vi "main_ctrl.vi"(8 "error in":errorcluster) -> (0 "error out":errorcluster caption="Error Out")   [LabVIEW 2013]
uses:
  <vilib>/Rock Robotics/WPI/DriverStation/WPI_DriverStationRobotMode2.ctl
  typedefs/fg_typedef.ctl
  <vilib>/Rock Robotics/WPI/Solenoid/WPI_SolenoidValue.ctl
  typedefs/subStates.ctl
  typedefs/singleUseSubstate.ctl
  typedefs/vision enable.ctl
  <vilib>/Rock Robotics/WPI/Compressor/WPI_CompressorGetSetRefNum.vi
  <vilib>/Rock Robotics/WPI/RobotDrive/WPI_RobotDriveGetSetRefNum.vi
  <vilib>/Rock Robotics/WPI/Solenoid/WPI_SolenoidGetEnum.vi
  <vilib>/Rock Robotics/WPI/Solenoid/WPI_SolenoidSetEnum.vi
  <vilib>/Rock Robotics/WPI/RobotDrive/WPI_RobotDriveArcadeDrive_Standard(NoSaturation).vi
  typedefs/vision data.ctl
panel:
  in  "Arcade Drive?":bool=TRUE
  out "Y Axis":dbl
  out "X Axis":dbl
  out "error In":errorcluster caption="Error In"
  out "Belts":dbl(knob) scale=-1.0..1.0
  out "Arm Encoder Rate":dbl(graph)
  out "Arm Encoder Distance":dbl(graph)
  out "Shifter State":cluster{"Shifted High":bool, "Shifted Low":bool}
  out "Extended":bool
  out "Retracted":bool
  out "Light Sensor":bool
  out "Belt Output":dbl
  out "Arm Distance":dbl
  out "Arm Rate":dbl
  in  "Joystick Override":bool
  in  "Joystick Y Manual":dbl(slide) scale=-1.0..1.0
  out "Left Drive Distance":dbl
  out "Right Drive Distance":dbl
  out "Left Drive Rate":dbl
  out "Right Drive Rate":dbl
  in  "Piston Actuation Commands":T1
  in  "Enables":T2
  out "Robot Mode":T3
  out "Vision SPI":u32
  out "Vision IPS":dbl
  out "Main IPS":dbl
  out "Main SPI":u32
  # "Inputs"
  # "Sensors"
  # "MAIN CONTROL"
  # "holds robot control code - dual parallel state machine"
  # "SPI: milliseconds per iteration\nIPS: iterations per second"
  # "Right Shooter Piston Sensors"
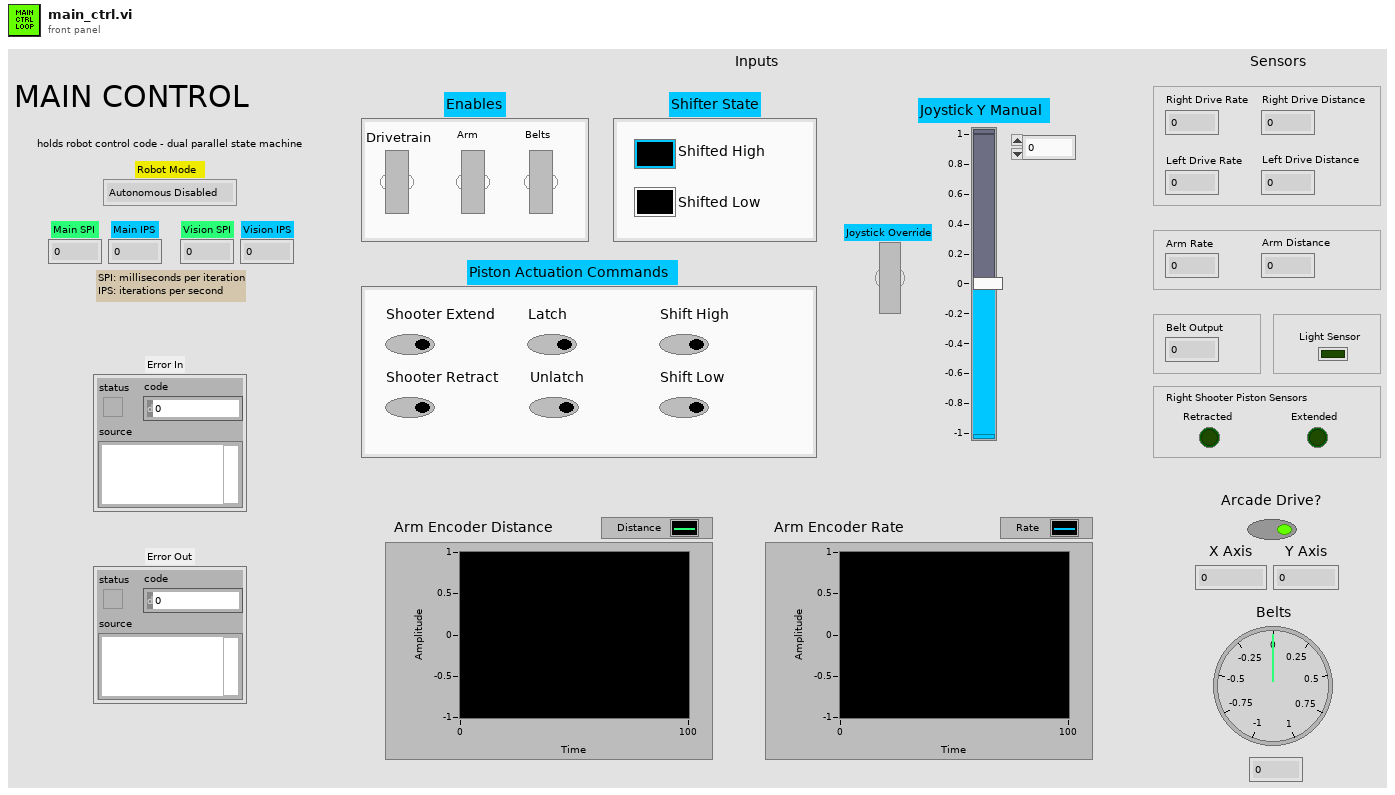
[diagram p1: front panel]
types:
  T1 = cluster{"Shooter Extend":bool, "Shooter Retract":bool, "Latch":bool, "Unlatch":bool, "Shift High":bool, "Shift Low":bool}
  T2 = cluster{"Drivetrain":bool, "Arm":bool, "Belts":bool}
  T3 = typedef "WPI_DriverStationRobotMode2.ctl" = enum16{"Autonomous Disabled", "Autonomous Enabled", "Teleop Disabled", "Teleop Enabled", "Timeout", "Finish", "Test Disabled", "Test Enabled"}
  T4 = typedef "WPI_RobotDriveDevRef.ctl" = cluster{"DevStatus":errorcluster, "Motors[]":T5[], "Square Inputs":bool, "Max Output":dbl, "Isochronous":bool}
  T5 = typedef "WPI_MotorControlDeviceRef.ctl" = cluster{"DeviceStatus":errorcluster, "Type":enum16{"PWM", "CAN"}, "PWM":cluster{"Digital Module":T6, "PWM Channel":T7, "DeadBand":T8}, "CAN":cluster{"Device Number":u8, "Control Mode":T9, "Semaphore":T10, "Max Vout":dbl}, "Invert":bool, "TransformRef":T11, "InvTransformRef":T11}
  T6 = typedef "FPGA_TypedefDigitalModule.ctl" = enum16{"Digital Module 1", "Digital Module 2"}
  T7 = typedef "FPGA_DIOPWMChannel.ctl" = enum8{"PWM 1", "PWM 2", "PWM 3", "PWM 4", "PWM 5", "PWM 6", "PWM 7", "PWM 8", "PWM 9", "PWM 10", "Invalid"}
  T8 = typedef "WPI_PWMDeadband.ctl" = cluster{"Name":string, "maxPositivePwm":i32, "minPositivePwm":i32, "centerPwm":i32, "maxNegativePwm":i32, "minNegativePwm":i32, "angularRange":u16}
  T9 = typedef "WPI_CANJaguar_ControlMode.ctl" = enum8{"Percent VBus", "Current", "Speed", "Position", "Voltage"}
  T10 = typedef "Semaphore RefNum" = refnum<k1>
  T11 = typedef "WPI_PWMTransform_ConPane.ctl" = refnum<vi>
  T12 = typedef "WPI_SolenoidDevRef.ctl" = cluster{"DevStatus":errorcluster, "Solenoid Module":T13, "Forward Solenoid Channel":T14, "Reverse Solenoid Channel":T14}
  T13 = typedef "FPGA_TypedefSolenoidModule.ctl" = enum16{"Solenoid Module 1", "Solenoid Module 2"}
  T14 = typedef "WPI_SolenoidChannel.ctl" = enum8{"Solenoid 1", "Solenoid 2", "Solenoid 3", "Solenoid 4", "Solenoid 5", "Solenoid 6", "Solenoid 7", "Solenoid 8", "Invalid"}
  T15 = typedef "WPI_CompressorDevRef.ctl" = cluster{"DevStatus":errorcluster, "DigitalInputDevRef":T16, "RelayDevRef":T18}
  T16 = typedef "WPI_DigitalInputDevRef.ctl" = cluster{"DevStatus":errorcluster, "DIO Channel":T17, "Digital Module":T6}
  T17 = typedef "FPGA_DIOChannel.ctl" = enum8{"DIO 1", "DIO 2", "DIO 3", "DIO 4", "DIO 5", "DIO 6", "DIO 7", "DIO 8", "DIO 9", "DIO 10", "DIO 11", "DIO 12", "DIO 13", "DIO 14", "Invalid"}
  T18 = typedef "WPI_RelayDevRef.ctl" = cluster{"DevStatus":errorcluster, "Relay Channel":T19, "Digital Module":T6, "Relay Direction":T20}
  T19 = typedef "FPGA_DIORelayChannel.ctl" = enum8{"Relay 1", "Relay 2", "Relay 3", "Relay 4", "Relay 5", "Relay 6", "Relay 7", "Relay 8", "Invalid"}
  T20 = typedef "WPI_RelayDirection.ctl" = enum16{"Both directions", "Forward only", "Reverse only"}
  T21 = typedef "vision data.ctl" = cluster{"x":dbl, "y":dbl, "area":dbl, "width":dbl, "height":dbl, "Hot Goal Present?":bool, "distance":dbl}
  T22 = typedef "vision enable.ctl" = enum16{"Enable", "Disable", "Stop"}
  T23 = typedef "fg_typedef.ctl" = enum16{"Get", "Set"}
  T24 = typedef "WPI_CameraDevRef.ctl" = cluster{"Camera Address":string, "CameraStatus":errorcluster, "Acquire Image Notifier":refnum<notifier>}
  T25 = typedef "IMAQ Image.ctl" = refnum<image>
  T26 = cluster{"Vision mSPI":u32, "Main mSPI":u32, "Dash mSPI":u32}
  T27 = typedef "WPI_SolenoidValue.ctl" = enum16{"Off", "On", "Forward", "Reverse"}
  T28 = typedef "singleUseSubstate.ctl" = enum16{"null", "wait", "shift high", "shift low"}
  T29 = cluster{"Joystick Y Manual":dbl, "Joystick Override":bool, "Piston Actuation Commands":cluster{"Shooter Extend":bool, "Shooter Retract":bool, "Latch Extend":bool, "Latch Retract":bool, "Shift High":bool, "Shift Low":bool}, "Enables":cluster{"Drivetrain":bool, "Arm":bool, "Belts":bool}}
  T30 = typedef "WPI_DriverStationDerivedRobotMode.ctl" = enum16{"Init", "Execute", "Stop"}
  T31 = typedef "subStates.ctl" = enum16{"null", "wait", "driver control", "auto", "manual override", "hold position", "rotate", "pickup", "pass", "load", "goto shoot", "shoot", "cancel", "end"}
  T32 = typedef "Loop 2 Datatype.ctl" = cluster{"State":T31, "Waiting Loop":i32, "State to Wait For":i32, "Loop ID":i32, "Exit Value":i32, "Joystick Y":dbl}
  T33 = typedef "Loop 1 Datatype.ctl" = cluster{"State":T31, "Waiting Loop":i32, "State to Wait For":i32, "Loop ID":i32, "Exit Value":i32}
  T34 = typedef "Loop 3 Datatype.ctl" = cluster{"State":T31, "Waiting Loop":i32, "State to Wait For":i32, "Loop ID":i32, "Exit Value":i32, "Joystick Y":dbl}
  T35 = typedef "Loop 0 Datatype.ctl" = cluster{"State":T31, "Waiting Loop":i32, "State to Wait For":i32, "Loop ID":i32, "Exit Value":i32, "X Axis":dbl, "Y Axis":dbl}
  T36 = typedef "Loop 4 Datatype.ctl" = cluster{"State":T31, "Waiting Loop":i32, "State to Wait For":i32, "Loop ID":i32, "Exit Value":i32}
  T37 = typedef "WPI_EncoderDevRef.ctl" = cluster{"DevStatus":errorcluster, "EncoderIndex":T38, "CounterIndex":T39, "DistancePerCount":dbl, "Decoding Type":T40}
  T38 = typedef "FPGA_EncoderIdx.ctl" = enum8{"Enc 0", "Enc 1", "Enc 2", "Enc 3", "Invalid"}
  T39 = typedef "FPGA_CounterCtrSystemIndex.ctl" = enum8{"Ctr 0", "Ctr 1", "Ctr 2", "Ctr 3", "Ctr 4", "Ctr 5", "Ctr 6", "Ctr 7", "Invalid"}
  T40 = typedef "WPI_EncoderType.ctl" = enum16{"1x", "2x", "4x"}
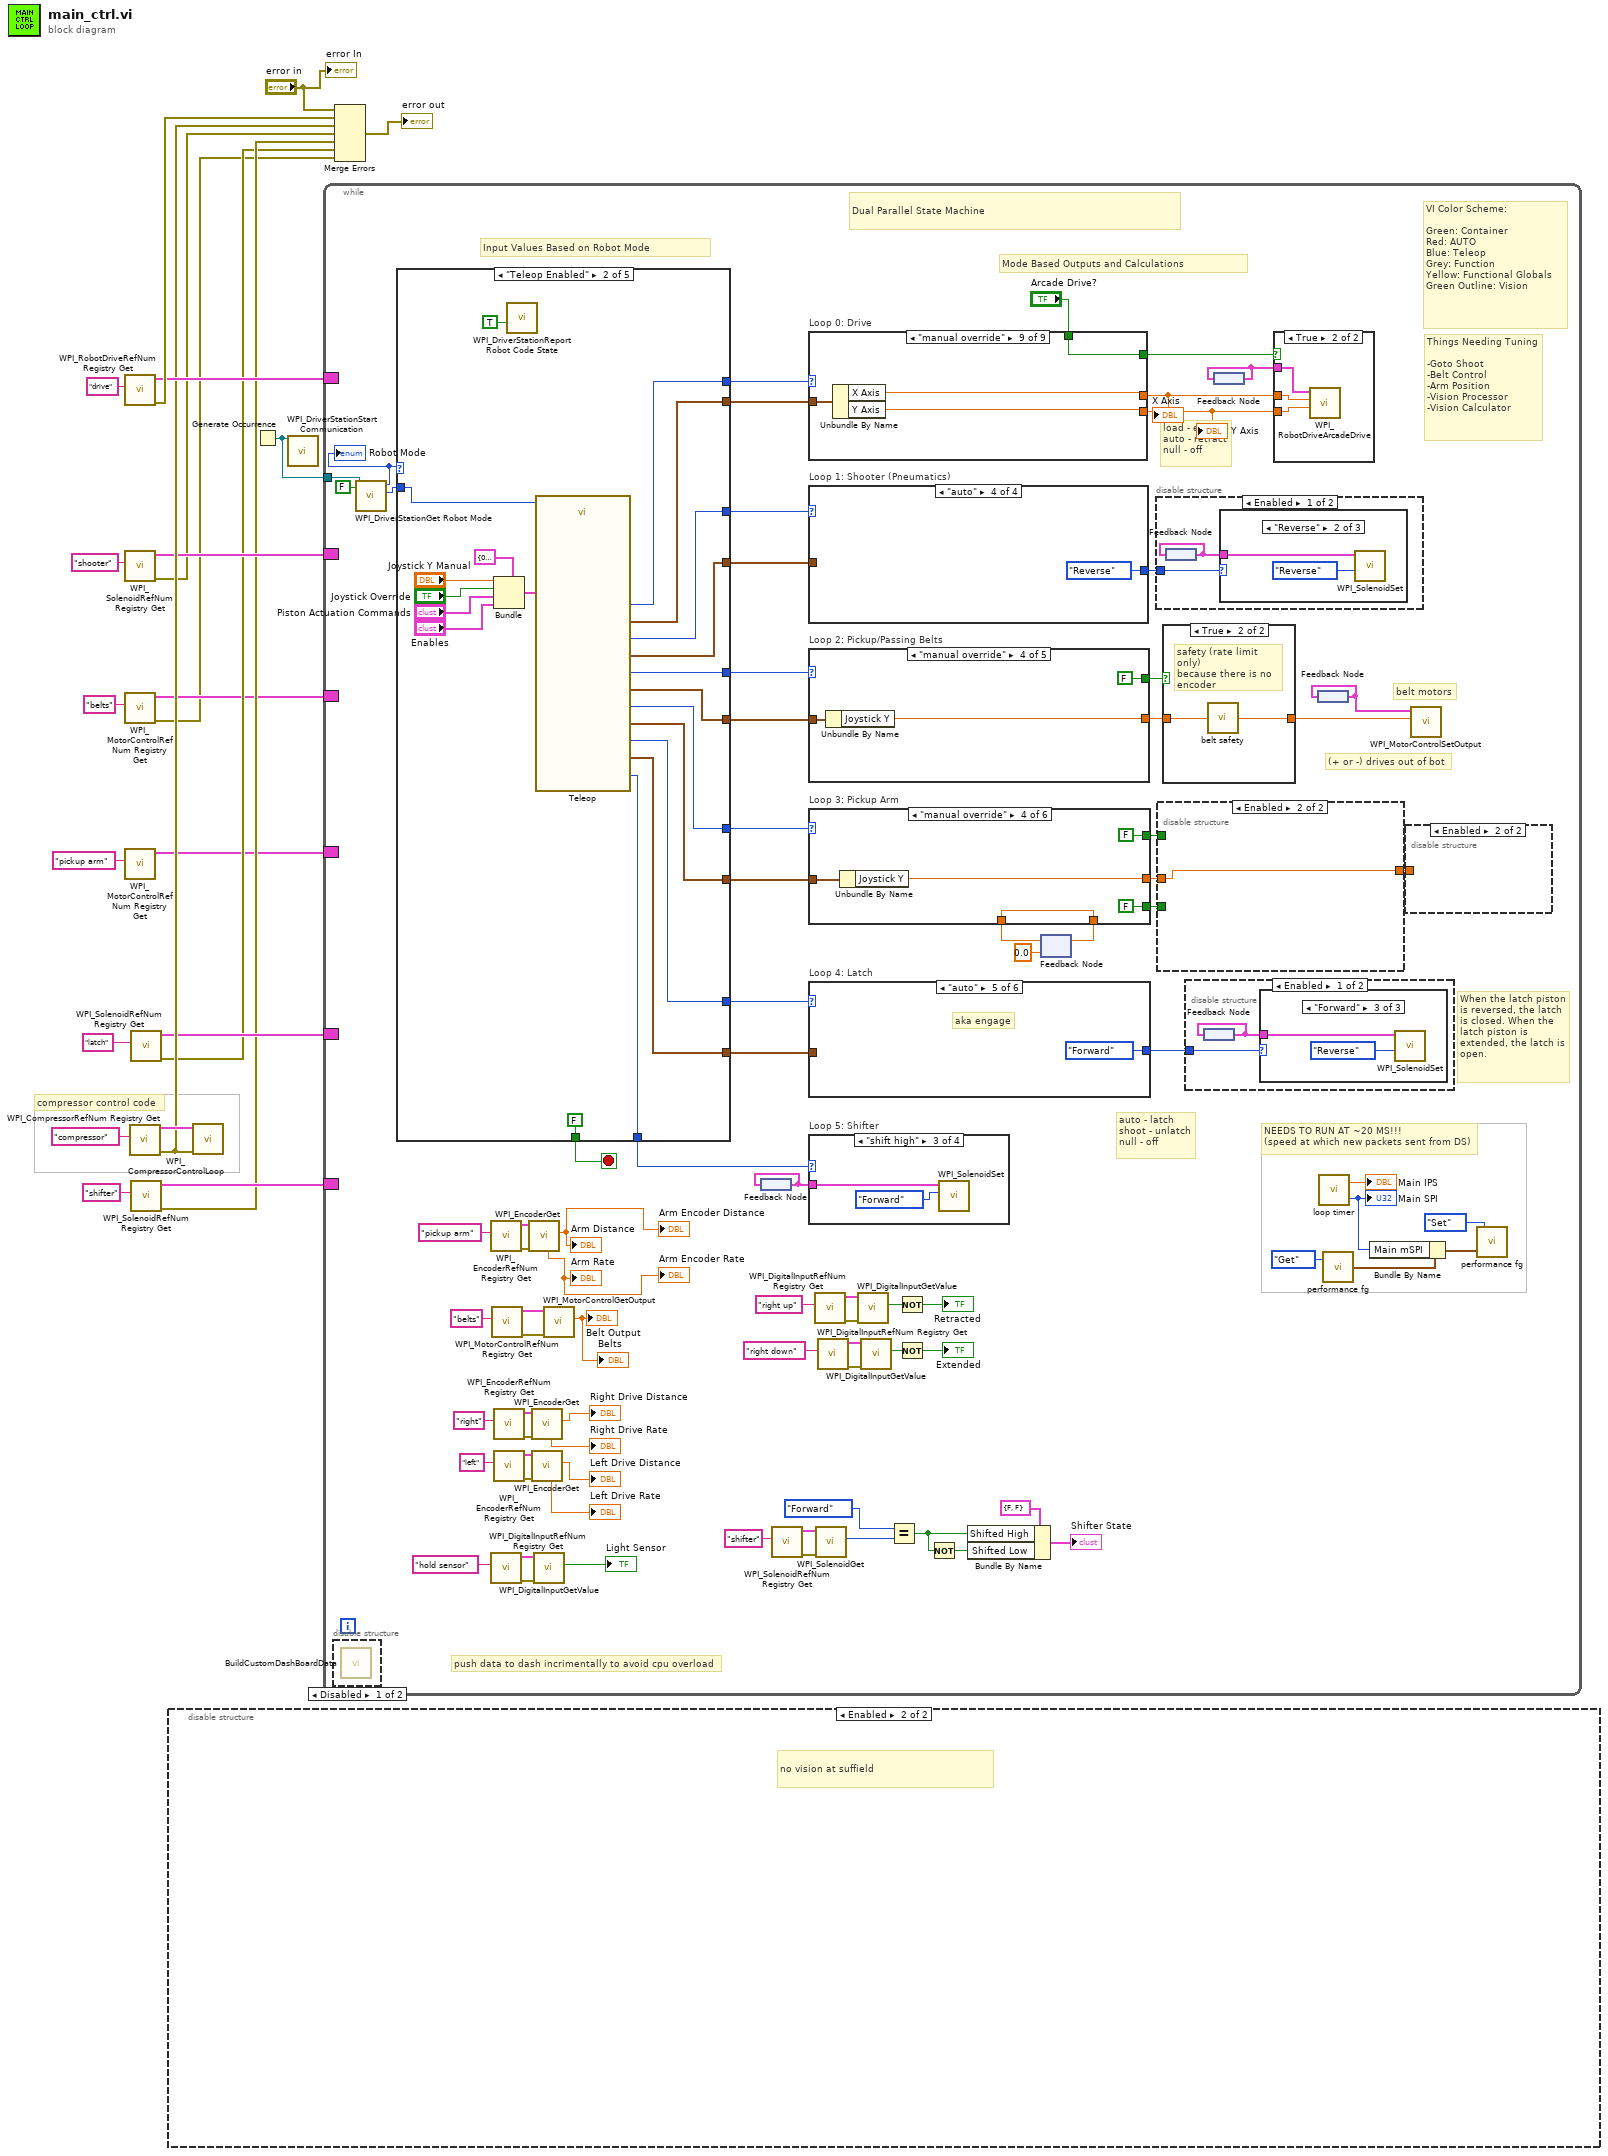
[diagram p0: block diagram]
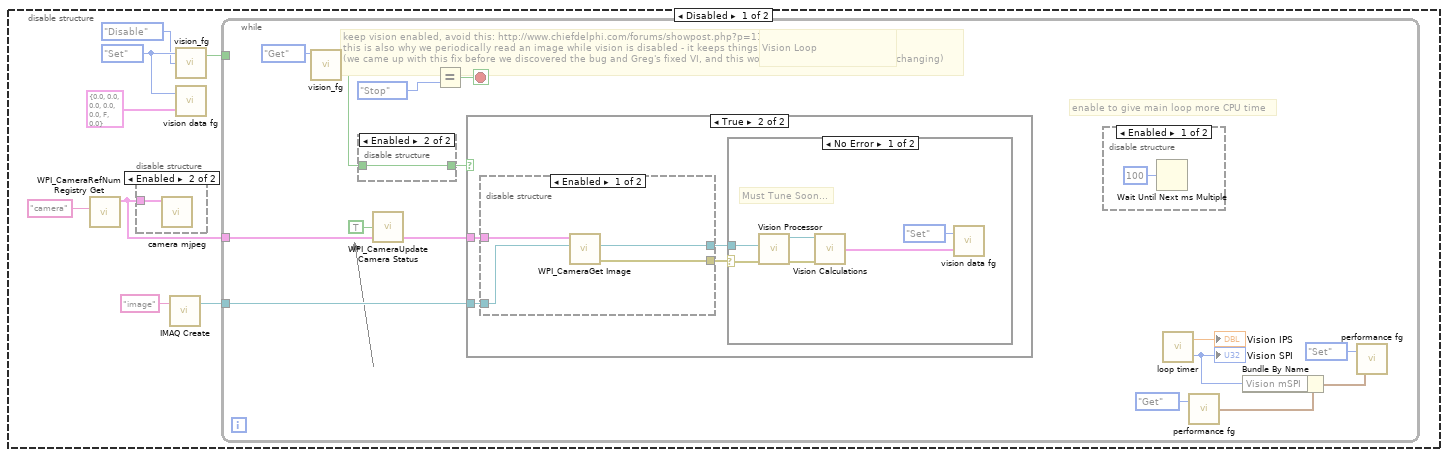
[diagram p2: hidden frame]
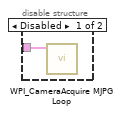
[diagram p3: hidden frame]
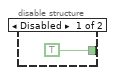
[diagram p4: hidden frame]
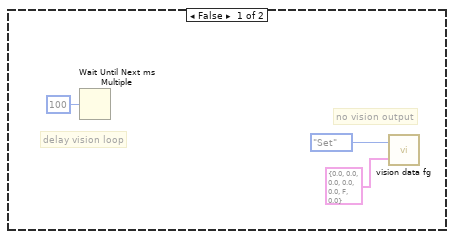
[diagram p6: hidden frame]
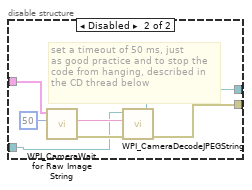
[diagram p8: hidden frame]
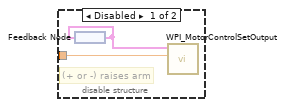
[diagram p10: hidden frame]
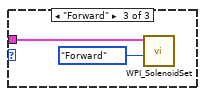
[diagram p12: hidden frame]
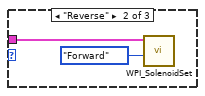
[diagram p15: hidden frame]
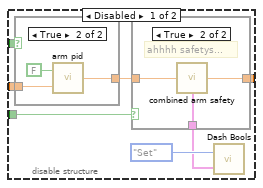
[diagram p17: hidden frame]
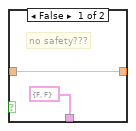
[diagram p18: hidden frame]
diagram:
  # "compressor control code"
  n1 = call <vilib>:"WPI_RobotDriveRefNum Registry Get.vi"("refnum name"="drive") -> ("error out"=w20:errorcluster, "RobotDriveDevRef"=w19:T4)  [unwired: 9 in]
  n2 = call <vilib>:"WPI_SolenoidRefNum Registry Get.vi"("refnum name"="shooter") -> ("error out"=w8:errorcluster, "SolenoidDevRef"=w12:T12)  [unwired: 9 in]
  n3 = call <vilib>:"WPI_MotorControlRefNum Registry Get.vi"("refnum name"="belts") -> ("error out"=w4:errorcluster, "MotorControlDevRef"=w6:T5)  [unwired: 9 in]
  n4 = call <vilib>:"WPI_MotorControlRefNum Registry Get.vi"("refnum name"="pickup arm") -> ("MotorControlDevRef"=w2:T5)  [unwired: 9 in, 1 out]
  n5 = call <vilib>:"WPI_CompressorRefNum Registry Get.vi"("refnum name"="compressor") -> ("error out"=w15:errorcluster, "CompressorDevRef"=w18:T15)  [unwired: 9 in]
  n6 = call <vilib>:"WPI_SolenoidRefNum Registry Get.vi"("refnum name"="latch") -> ("error out"=w7:errorcluster, "SolenoidDevRef"=w10:T12)  [unwired: 9 in]
  n7 = call <vilib>:"WPI_SolenoidRefNum Registry Get.vi"("refnum name"="shifter") -> ("error out"=w9:errorcluster, "SolenoidDevRef"=w17:T12)  [unwired: 9 in]
  n8 = disable-structure shown="Enabled" {
    frame Disabled {
      w29 = fg_typedef."Set" ("Enum")
      n9 = call <vilib>:"WPI_CameraRefNum Registry Get.vi"("refnum name"="camera") -> ("CameraDevRef"=w26:T24)  [unwired: 9 in, 1 out]
      n10 = disable-structure shown="Enabled" {
        disable-tunnel: w26 -> [w32 w33]
        frame Disabled {
          n11 = call <vilib>:"WPI_CameraAcquire MJPG Loop.vi"("CameraDevRef"=w32) -> ()  [unwired: 11 in]
        }
        frame Enabled {
          n12 = call "camera mjpeg.vi"("CameraDevRef"=w33) -> ()  [unwired: 11 in]
        }
      }
      n13 = call "IMAQ Create"("Image Name"="image") -> ("New Image"=w31:T25)  [unwired: 4 in, 1 out]
      n14 = call "vision_fg.vi"("Action"=vision_enable."Disable", "Menu"=w29) -> ("Enabled?"=w30:bool)  [unwired: 1 in, 1 out]
      n15 = call "vision data fg.vi"("Input"=T21 {"x"=0.0, "y"=0.0, "area"=0.0, "width"=0.0, "height"=0.0, "Hot Goal Present?"=FALSE, "distance"=0.0} ("Cluster"), "Menu"=w29) -> ()  [unwired: 1 out]
      n16 = while {
        tunnel: w31 -> [w48]
        tunnel: w26 -> [w47]
        tunnel: w30 -> [_]
        stop <- w49 stop-if-true
        # "keep vision enabled, avoid this: http://www.chiefdelphi.com/forums/showpost.php?p=1128407&postcount=2\nthis is also why we periodically read an image while vision is disabled - it keeps things from timing out\n(we came up with this fix before we discovered the bug and Greg's fixed VI, and this worked well, so it wasn't worth changing)"
        # "enable to give main loop more CPU time"
        # "Vision Loop"
        n17 = call "vision_fg.vi"("Menu"=fg_typedef."Get" ("Enum")) -> ("State Out"=w43:T22, "Enabled?"=w34:bool)  [unwired: 2 in]
        n18 = disable-structure shown="Enabled" {
          disable-tunnel: [TRUE w51] -> w35
          disable-tunnel: w34 -> [_ w51]
          frame Disabled {
          }
          frame Enabled {
          }
        }
        n19 = call <vilib>:"WPI_CameraUpdate Camera Status.vi"("CameraDevRef In"=w47, "Enable Vision"=TRUE) -> ("CameraDevRef Out"=w46:T24)  [unwired: 3 in]
        n20 = Equal?(x=w43, y=vision_enable."Stop") -> (x = y?=w49:bool)
        n21 = case shown="True" w35 {
          tunnel: w48 -> [_ w59]
          tunnel: w46 -> [_ w58]
          frame False {
            # "no vision output"
            # "delay vision loop"
            n22 = Wait Until Next ms Multiple(millisecond multiple=u32 100) -> ()  [unwired: 1 out]
            n23 = call "vision data fg.vi"("Input"=T21 {"x"=0.0, "y"=0.0, "area"=0.0, "width"=0.0, "height"=0.0, "Hot Goal Present?"=FALSE, "distance"=0.0} ("Cluster"), "Menu"=fg_typedef."Set" ("Enum")) -> ()  [unwired: 1 out]
          }
          frame True {
            n24 = disable-structure shown="Enabled" {
              disable-tunnel: w59 -> [w68 w72]
              disable-tunnel: w58 -> [w69 w74]
              disable-tunnel: [w67 w71] -> w57
              disable-tunnel: [w66 w70] -> w56
              frame Enabled {
                n25 = call <vilib>:"WPI_CameraGet Image.vi"("Image"=w68, "CameraDevRef"=w69) -> ("error out"=w66:errorcluster, "Image Out"=w67:T25)  [unwired: 7 in, 1 out]
              }
              frame Disabled {
                # "set a timeout of 50 ms, just\nas good practice and to stop the \ncode from hanging, described in \nthe CD thread below"
                n26 = call <vilib>:"WPI_CameraWait for Raw Image String.vi"("Timeout in ms (-1)"=50, "CameraDevRef"=w74) -> ("error out"=w76:errorcluster, "String"=w75:string)  [unwired: 3 in, 5 out]
                n27 = call <vilib>:"WPI_CameraDecodeJPEGString.vi"("error in"=w76, "Compressed Image"=w75, "Image In"=w72) -> ("error out"=w70:errorcluster, "Image Out"=w71:T25)  [unwired: 3 out]
              }
            }
            n28 = case shown="No Error" w56 {
              selector: w56 -> [w64 _]
              tunnel: w57 -> [w63 _]
              frame No Error {
                # "Must Tune Soon..."
                n29 = call "Vision Processor.vi"("error in"=w64, "Image In"=w63) -> ("error out"=w61:errorcluster, "Image Out"=w62:T25)  [unwired: 5 in]
                n30 = call "Vision Calculations.vi"("Image In"=w62, "error in"=w61) -> ("Vision Data"=w60:T21)  [unwired: 3 in]
                n31 = call "vision data fg.vi"("Input"=w60, "Menu"=fg_typedef."Set" ("Enum")) -> ()  [unwired: 1 out]
              }
              frame Error {
              }
            }
          }
        }
        n32 = disable-structure shown="Enabled" {
          frame Enabled {
            n33 = Wait Until Next ms Multiple(millisecond multiple=u32 100) -> ()  [unwired: 1 out]
          }
          frame Disabled {
          }
        }
        n34 = call "loop timer.vi"() -> ("IPS"=→"Vision IPS":dbl, "SPI"=w41:u32)  [unwired: 1 in]
        "Vision SPI" <- w41
        n35 = call "performance fg.vi"("Menu"=fg_typedef."Get") -> ("Output"=w39:T26)  [unwired: 1 in]
        n36 = Bundle By Name(cluster=w39, "Vision mSPI"=w41) -> (w38:T26)
        n37 = call "performance fg.vi"("Input"=w38, "Menu"=fg_typedef."Set") -> ()  [unwired: 1 out]
      }
    }
    frame Enabled {
      # "no vision at suffield"
    }
  }
  n38 = call <vilib>:"WPI_CompressorControlLoop.vi"("error in (no error)"=w15, "CompressorDevRef"=w18) -> ()  [unwired: 10 in]
  n39 = Generate Occurrence() -> (w14:refnum<k4>)
  n40 = call <vilib>:"WPI_DriverStationStart Communication.vi"("occurrence"=w14) -> ()  [unwired: 11 in]
  n41 = while {
    tunnel: w14 -> [w82]
    border: w19 -> [_]
    border: w17 -> [_]
    border: w12 -> [_]
    border: w10 -> [_]
    border: w6 -> [_]
    border: w2 -> [_]
    stop <- w156 stop-if-true
    # "belt motors"
    # "auto - latch\nshoot - unlatch\nnull - off"
    # "load - extend\nauto - retract\nnull - off"
    # "When the latch piston\nis reversed, the latch\nis closed. When the\nlatch piston is\nextended, the latch is\nopen."
    # "push data to dash incrimentally to avoid cpu overload"
    # "Things Needing Tuning\n\n-Goto Shoot\n-Belt Control\n-Arm Position\n-Vision Processor\n-Vision Calculator"
    # "(+ or -) drives out of bot"
    # "VI Color Scheme:\n\nGreen: Container\nRed: AUTO\nBlue: Teleop\nGrey: Function\nYellow: Functional Globals\nGreen Outline: Vision"
    # "Input Values Based on Robot Mode"
    # "Mode Based Outputs and Calculations"
    # "NEEDS TO RUN AT ~20 MS!!!\n(speed at which new packets sent from DS)"
    # "Dual Parallel State Machine"
    n42 = disable-structure shown="Disabled" {
      frame Disabled {
        n43 = call "BuildCustomDashBoardData.vi"() -> ()  [unwired: 12 in]
      }
      frame Enabled {
      }
    }
    n44 = call <vilib>:"WPI_DriverStationGet Robot Mode.vi"("Finish"=FALSE, "DS Occurrence"=w82) -> ("Call Context"=w80:T30, "Robot Mode"=w81:T3)  [unwired: 8 out]
    "Robot Mode" <- w81
    n45 = case shown="\"Teleop Enabled\"" w81 {
      tunnel: [w369 w406 w408 w414 w420] -> w137
      tunnel: w80 -> [w360 w402 _ _ _]
      tunnel: [w367 w405 w408 w414 w420] -> w158
      tunnel: [w361 w403 singleUseSubstate."null" ("SubState 5") singleUseSubstate."null" ("SubState 5") singleUseSubstate."null" ("SubState 5")] -> w157
      tunnel: [FALSE FALSE FALSE FALSE TRUE] -> w156
      tunnel: [w371 w401 w408 w414 w420] -> w149
      tunnel: [w370 w400 _ _ _] -> w150
      tunnel: [w368 w399 _ _ _] -> w148
      tunnel: [w366 w398 _ _ _] -> w147
      tunnel: [w364 w397 _ _ _] -> w145
      tunnel: [w362 w396 _ _ _] -> w144
      tunnel: [w363 w395 w408 w414 w420] -> w143
      tunnel: [w365 w394 w408 w414 w420] -> w142
      frame "Autonomous Enabled" {
        n46 = disable-structure shown="Enabled" {
          disable-tunnel: [w384 w386] -> w371
          disable-tunnel: [w383 _] -> w370
          disable-tunnel: [w382 w386] -> w369
          disable-tunnel: [w381 _] -> w368
          disable-tunnel: [w380 w386] -> w367
          disable-tunnel: [w379 _] -> w366
          disable-tunnel: [w378 w386] -> w365
          disable-tunnel: [w377 _] -> w364
          disable-tunnel: [w376 w386] -> w363
          disable-tunnel: [w375 _] -> w362
          disable-tunnel: [w374 singleUseSubstate."null" ("SubState 5")] -> w361
          disable-tunnel: w360 -> [w373 _]
          frame Disabled {
            n47 = call "Autonomous.vi"("Call Context"=w373) -> ("SubState 2"=w380:T31, "Loop 2 Data"=w379:T32, "SubState 1"=w382:T31, "Loop 1 Data"=w381:T33, "Loop 3 Data"=w377:T34, "SubState 0"=w384:T31, "SubState 3"=w378:T31, "Loop 0 Data"=w383:T35, "Loop 4 Data"=w375:T36, "SubState 4"=w376:T31, "SubState 5"=w374:T28)
          }
          frame Enabled {
            w386 = subStates."null" ("SubState 0")
          }
        }
        n48 = call <vilib>:"WPI_DriverStationReport Robot Code State.vi"("Autonomous"=TRUE) -> ()  [unwired: 10 in, 1 out]
      }
      frame "Teleop Enabled" {
        n49 = Bundle(cluster=T29 {"Joystick Y Manual"=0.0, "Joystick Override"=FALSE, "Piston Actuation Commands"={"Shooter Extend"=FALSE, "Shooter Retract"=FALSE, "Latch Extend"=FALSE, "Latch Retract"=FALSE, "Shift High"=FALSE, "Shift Low"=FALSE}, "Enables"={"Drivetrain"=FALSE, "Arm"=FALSE, "Belts"=FALSE}}, "Joystick Y Manual"="Joystick Y Manual", "Joystick Override"="Joystick Override", "Piston Actuation Commands"="Piston Actuation Commands", "Enables"="Enables") -> (w391:T29)
        n50 = call <vilib>:"WPI_DriverStationReport Robot Code State.vi"("TeleOp"=TRUE) -> ()  [unwired: 10 in, 1 out]
        n51 = call "Teleop.vi"("Call Context"=w402, "Input"=w391) -> ("SubState 3"=w394:T31, "SubState 4"=w395:T31, "SubState 5"=w403:T28, "Loop 3 Data"=w397:T34, "Loop 4 Data"=w396:T36, "SubState 0"=w401:T31, "Loop 1 Data"=w399:T33, "Loop 0 Data"=w400:T35, "SubState 1"=w406:T31, "Loop 2 Data"=w398:T32, "SubState 2"=w405:T31)  [unwired: 7 in]
      }
      frame "Autonomous Disabled", "Teleop Disabled", "Timeout" {
        w408 = subStates."null" ("SubState 0")
        # "set all loops to null"
        # "make sure to disable vision\nwe don't need it here"
        # "robot disabled, timeout"
        n52 = call <vilib>:"WPI_DriverStationReport Robot Code State.vi"("Disabled"=TRUE) -> ()  [unwired: 10 in, 1 out]
        n53 = call "vision_fg.vi"("Action"=vision_enable."Disable", "Menu"=fg_typedef."Set") -> ()  [unwired: 1 in, 2 out]
      }
      frame "Test Disabled", "Test Enabled" {
        w414 = subStates."null" ("SubState 0")
        # "set all loops to null"
        # "make sure to disable vision\nwe don't need it here"
        # "test, unused"
        n54 = call <vilib>:"WPI_DriverStationReport Robot Code State.vi"("Test"=TRUE) -> ()  [unwired: 10 in, 1 out]
        n55 = call "vision_fg.vi"("Action"=vision_enable."Disable", "Menu"=fg_typedef."Set") -> ()  [unwired: 1 in, 2 out]
      }
      frame "Finish" {
        w420 = subStates."end"  # Stop All Loops
        # "stop the while loop"
        # "stop DS comms"
        # "stop vision loop"
        n56 = call <vilib>:"WPI_DriverStationStop Communication.vi"("StopCommunication"=TRUE) -> ()  [unwired: 10 in, 1 out]
        n57 = call "vision_fg.vi"("Action"=vision_enable."Stop", "Menu"=fg_typedef."Set") -> ()  [unwired: 1 in, 2 out]
      }
    }
    n58 = call <vilib>:"WPI_EncoderRefNum Registry Get.vi"("refnum name"="pickup arm") -> ("error out"=w119:errorcluster, "EncoderDevRef"=w120:T37)  [unwired: 9 in]
    n59 = call <vilib>:"WPI_DigitalInputRefNum Registry Get.vi"("refnum name"="hold sensor") -> ("error out"=w106:errorcluster, "DigitalInputDevRef"=w107:T16)  [unwired: 9 in]
    n60 = call <vilib>:"WPI_MotorControlRefNum Registry Get.vi"("refnum name"="belts") -> ("error out"=w124:errorcluster, "MotorControlDevRef"=w123:T5)  [unwired: 9 in]
    n61 = call <vilib>:"WPI_EncoderRefNum Registry Get.vi"("refnum name"="right") -> ("error out"=w118:errorcluster, "EncoderDevRef"=w117:T37)  [unwired: 9 in]
    n62 = call <vilib>:"WPI_EncoderRefNum Registry Get.vi"("refnum name"="left") -> ("error out"=w113:errorcluster, "EncoderDevRef"=w114:T37)  [unwired: 9 in]
    n63 = call <vilib>:"WPI_EncoderGet.vi"("error in (no error)"=w119, "EncoderDevRef"=w120) -> ("Distance"=→"Arm Distance" →"Arm Encoder Distance":dbl, "Rate"=→"Arm Rate" →"Arm Encoder Rate":dbl)  [unwired: 4 in, 4 out]
    n64 = call <vilib>:"WPI_EncoderGet.vi"("error in (no error)"=w118, "EncoderDevRef"=w117) -> ("Distance"=→"Right Drive Distance":dbl, "Rate"=→"Right Drive Rate":dbl)  [unwired: 4 in, 4 out]
    n65 = call <vilib>:"WPI_EncoderGet.vi"("error in (no error)"=w113, "EncoderDevRef"=w114) -> ("Distance"=→"Left Drive Distance":dbl, "Rate"=→"Left Drive Rate":dbl)  [unwired: 4 in, 4 out]
    n66 = call <vilib>:"WPI_DigitalInputGetValue.vi"("error in (no error)"=w106, "DigitalInputDevRef"=w107) -> ("Value"=→"Light Sensor":bool)  [unwired: 7 in, 2 out]
    n67 = call <vilib>:"WPI_MotorControlGetOutput.vi"("error in (no error)"=w124, "MotorControlDevRef"=w123) -> ("Output"=→"Belt Output" →"Belts":dbl)  [unwired: 7 in, 2 out]
    n68 = feedback #1() -> (w146:T12)
    n69 = feedback-in #1(w146) -> ()
    n70 = call <vilib>:"WPI_SolenoidRefNum Registry Get.vi"("refnum name"="shifter") -> ("error out"=w91:errorcluster, "SolenoidDevRef"=w90:T12)  [unwired: 9 in]
    n71 = case "Loop 0: Drive" shown="\"manual override\"" w149 {
      tunnel: w150 -> [w202 w206 w218 w225 w242 w249 _ _ w263]
      tunnel: [w200 w204 w216 w227 w239 w251 w254 w259 w262] -> w140
      tunnel: [w200 w204 w215 w226 w238 w250 w253 w259 w261] -> w139
      tunnel: [FALSE FALSE TRUE FALSE FALSE FALSE FALSE FALSE w260] -> w141
      tunnel: "Arcade Drive?" -> [_ _ _ _ _ _ _ _ w260]
      frame "null", Default {
        w200 = 0.0 ("X Axis")
        n72 = Unbundle By Name(w202) -> ("Loop ID"=w203:i32)
        n73 = call "null.vi"("This Loop ID"=w203) -> ()  [unwired: 2 in]
      }
      frame "wait" {
        w204 = 0.0 ("X Axis")
        n74 = Unbundle By Name(w206) -> ("Loop ID"=w210:i32, "Exit Value"=w209:i32, "Waiting Loop"=w208:i32, "State to Wait For"=w207:i32)
        n75 = call "wait.vi"("State to wait for"=w207, "Waiting Loop ID"=w208, "time (ms)"=w209, "Current Loop ID"=w210) -> ()  [unwired: 1 out]
      }
      frame "driver control" {
        # "filter joysticks"
        n76 = Unbundle By Name(w218) -> ("X Axis"=w211:dbl, "Y Axis"=w214:dbl)
        n77 = call "Joystick Error Filter.vi"("Axis"=w211) -> ("Filtered Axis"=w212:dbl)
        n78 = call "Joystick Error Filter.vi"("Axis"=w214) -> ("Filtered Axis"=w213:dbl)
        n79 = disable-structure shown="Enabled" {
          disable-tunnel: w212 -> [w222 w224]
          disable-tunnel: w213 -> [w221 w223]
          disable-tunnel: [w220 w224] -> w216
          disable-tunnel: [w219 w223] -> w215
          frame Disabled {
            n80 = call "calc arcade drive pwm.vi"("Y axis value"=w221, "X axis value"=w222) -> ("Right Speed"=w219:dbl, "Left Speed"=w220:dbl)  [unwired: 1 in, 1 out]
          }
          frame Enabled {
          }
        }
      }
      frame "auto" {
        n81 = disable-structure shown="Enabled" {
          disable-tunnel: [w236 _] -> w227
          disable-tunnel: [w235 _] -> w226
          disable-tunnel: w225 -> [w231 _]
          frame Disabled {
            n82 = Unbundle By Name(w231) -> ("Z Axis"=w229:dbl)
            n83 = call "Vision Tracking X.vi"("Tweak"=w229) -> ("right speed"=w230:dbl, "left speed"=w233:dbl)
            n84 = call "closed drive.vi"("Acrade Drive?"=FALSE, "Y axis value (Left)"=w233, "X axis value (Right)"=w230, "Threshold (.4)"=0.0 ("Threshold")) -> ("right"=w235:dbl, "left"=w236:dbl)
          }
          frame Enabled {
            # "rotates toward target"
            # "not in use this year"
          }
        }
      }
      frame "hold position" {
        n85 = Unbundle By Name(w242) -> ("X Axis"=w241:dbl, "Y Axis"=w240:dbl)
        n86 = call "closed drive.vi"("Acrade Drive?"=TRUE, "Y axis value (Left)"=w240, "X axis value (Right)"=w241) -> ("right"=w238:dbl, "left"=w239:dbl)  [unwired: 1 in]
      }
      frame "rotate" {
        # "use these to carry actual information because this is\nfor autonomous only so there will not be joystick input"
        n87 = Unbundle By Name(w249) -> ("X Axis"=w248:dbl, "Y Axis"=w247:dbl)
        n88 = call "rotate.vi"("Angle"=w248, "Rate"=w247) -> ("finished?"=w244:bool, "left speed"=w251:dbl, "right speed"=w250:dbl)
        n89 = call "states FG.vi"("exit in"=w244, "menu (get)"=enum16{"set", "get"}."set", "Loop ID"=0) -> ()  [unwired: 5 in, 4 out]
      }
      frame "goto shoot" {
        # "consider implimenting closed hold with drive"
        n90 = call "vision data fg.vi"("Menu"=fg_typedef."Get") -> ("Output"=w255:T21)  [unwired: 1 in]
        n91 = call "goto location.vi"("Image Data"=w255) -> ("left speed"=w254:dbl, "right speed"=w253:dbl)
      }
      frame "end" {
        w259 = 0.0 ("X Axis")
      }
      frame "manual override" {
        n92 = Unbundle By Name(w263) -> ("X Axis"=w262:dbl, "Y Axis"=w261:dbl)
      }
    }
    "X Axis" <- w140
    "Y Axis" <- w139
    n93 = case "Loop 1: Shooter (Pneumatics)" shown="\"auto\"" w137 {
      tunnel: w148 -> [w349 w352 _ _]
      tunnel: [WPI_SolenoidValue."Off" ("Value") WPI_SolenoidValue."Off" ("Value") WPI_SolenoidValue."Forward" ("Value") WPI_SolenoidValue."Reverse" ("Value")] -> w125
      frame "null", Default {
        n94 = Unbundle By Name(w349) -> ("Loop ID"=w350:i32)
        n95 = call "null.vi"("This Loop ID"=w350) -> ()  [unwired: 2 in]
      }
      frame "wait" {
        n96 = Unbundle By Name(w352) -> ("Loop ID"=w356:i32, "Exit Value"=w355:i32, "Waiting Loop"=w354:i32, "State to Wait For"=w353:i32)
        n97 = call "wait.vi"("State to wait for"=w353, "Waiting Loop ID"=w354, "time (ms)"=w355, "Current Loop ID"=w356) -> ()  [unwired: 1 out]
      }
      frame "load" {
      }
      frame "auto" {
      }
    }
    n98 = case "Loop 2: Pickup/Passing Belts" shown="\"manual override\"" w158 {
      tunnel: w147 -> [w326 w329 w337 w340 w343]
      tunnel: [0.0 ("output") 0.0 ("output") w335 w338 w342] -> w131
      tunnel: [FALSE FALSE TRUE FALSE TRUE] -> w132
      frame "null", Default {
        n99 = Unbundle By Name(w326) -> ("Loop ID"=w325:i32)
        n100 = call "null.vi"("This Loop ID"=w325) -> ()  [unwired: 2 in]
      }
      frame "wait" {
        n101 = Unbundle By Name(w329) -> ("Loop ID"=w333:i32, "Exit Value"=w332:i32, "Waiting Loop"=w331:i32, "State to Wait For"=w330:i32)
        n102 = call "wait.vi"("State to wait for"=w330, "Waiting Loop ID"=w331, "time (ms)"=w332, "Current Loop ID"=w333) -> ()  [unwired: 1 out]
      }
      frame "driver control" {
        n103 = Unbundle By Name(w337) -> ("Joystick Y"=w334:dbl)
        n104 = call "Joystick Error Filter.vi"("Axis"=w334) -> ("Filtered Axis"=w335:dbl)
      }
      frame "manual override" {
        n105 = Unbundle By Name(w340) -> ("Joystick Y"=w338:dbl)
      }
      frame "pickup".."load", "cancel" {
        # "pickup, pass, load, and cancel"
        n106 = disable-structure shown="Disabled" {
          disable-tunnel: w343 -> [w347 _]
          disable-tunnel: [w344 _] -> w342
          frame Disabled {
            n107 = Unbundle By Name(w347) -> ("Tune Speed"=w346:dbl, "State"=w345:T31)
            n108 = call "belt control.vi"("State"=w345, "Joystick Z"=w346) -> ("output"=w344:dbl)
          }
          frame Enabled {
          }
        }
      }
    }
    n109 = case "Loop 4: Latch" shown="\"auto\"" w143 {
      tunnel: w144 -> [w266 w268 _ _ _ _]
      tunnel: [WPI_SolenoidValue."Off" ("Value") WPI_SolenoidValue."Off" ("Value") WPI_SolenoidValue."Off" ("Value") w274 WPI_SolenoidValue."Forward" ("Value") WPI_SolenoidValue."Reverse" ("Value")] -> w126
      frame "null", Default {
        n110 = Unbundle By Name(w266) -> ("Loop ID"=w265:i32)
        n111 = call "null.vi"("This Loop ID"=w265) -> ()  [unwired: 2 in]
      }
      frame "wait" {
        n112 = Unbundle By Name(w268) -> ("Loop ID"=w272:i32, "Exit Value"=w271:i32, "Waiting Loop"=w270:i32, "State to Wait For"=w269:i32)
        n113 = call "wait.vi"("State to wait for"=w269, "Waiting Loop ID"=w270, "time (ms)"=w271, "Current Loop ID"=w272) -> ()  [unwired: 1 out]
      }
      frame "driver control" {
      }
      frame "shoot" {
        # "aka disengage latch"
        n114 = disable-structure shown="Enabled" {
          disable-tunnel: [w278 WPI_SolenoidValue."Reverse" ("Value")] -> w274
          frame Disabled {
            n115 = call "latch shoot.vi"() -> ("Latch"=w277:T27, "Met Requierments for shooting?"=w275:bool)
            n116 = call "safe shoot error.vi"("Can Shoot Safely?"=w275, "Menu"=fg_typedef."Set") -> ()  [unwired: 1 out]
            n117 = call "re-init on shoot.vi"("Relay Value"=w277) -> ("Value"=w278:T27)
          }
          frame Enabled {
          }
        }
      }
      frame "auto" {
        # "aka engage"
      }
      frame "manual override" {
        # "unsafely shoot"
      }
    }
    n118 = case "Loop 5: Shifter" shown="\"shift high\"" w157 {
      tunnel: w146 -> [_ _ w320 w321]
      frame "null", Default {
      }
      frame "wait" {
      }
      frame "shift high" {
        n119 = call-poly <vilib>:"WPI_SolenoidSet.vi"("Value"=WPI_SolenoidValue."Forward", "SolenoidDevRef"=w320) -> ()  [unwired: 8 in, 2 out]
      }
      frame "shift low" {
        n120 = call-poly <vilib>:"WPI_SolenoidSet.vi"("Value"=WPI_SolenoidValue."Reverse", "SolenoidDevRef"=w321) -> ()  [unwired: 8 in, 2 out]
      }
    }
    n121 = call <vilib>:"WPI_DigitalInputRefNum Registry Get.vi"("refnum name"="right up") -> ("error out"=w104:errorcluster, "DigitalInputDevRef"=w103:T16)  [unwired: 9 in]
    n122 = call-poly <vilib>:"WPI_SolenoidGet.vi"("error in (no error)"=w91, "SolenoidDevRef"=w90) -> ("Value"=w89:T27)  [unwired: 7 in, 2 out]
    n123 = call <vilib>:"WPI_DigitalInputRefNum Registry Get.vi"("refnum name"="right down") -> ("error out"=w99:errorcluster, "DigitalInputDevRef"=w100:T16)  [unwired: 9 in]
    n124 = call <vilib>:"WPI_DigitalInputGetValue.vi"("error in (no error)"=w104, "DigitalInputDevRef"=w103) -> ("Value"=w98:bool)  [unwired: 7 in, 2 out]
    n125 = call <vilib>:"WPI_DigitalInputGetValue.vi"("error in (no error)"=w99, "DigitalInputDevRef"=w100) -> ("Value"=w97:bool)  [unwired: 7 in, 2 out]
    n126 = Equal?(x=WPI_SolenoidValue."Forward", y=w89) -> (x = y?=w87:bool)
    n127 = Not(x=w98) -> (.not. x?=→"Retracted":bool)
    n128 = Not(x=w97) -> (.not. x?=→"Extended":bool)
    n129 = Not(x=w87) -> (.not. x?=w86:bool)
    n130 = Bundle By Name(cluster=cluster{"Shifted High":bool, "Shifted Low":bool} {"Shifted High"=FALSE, "Shifted Low"=FALSE} ("Shifter State"), "Shifted High"=w87, "Shifted Low"=w86) -> (→"Shifter State":cluster{"Shifted High":bool, "Shifted Low":bool})
    n131 = feedback #2(0.0 ("setpoint")) -> (w128:dbl)
    n132 = case "Loop 3: Pickup Arm" shown="\"manual override\"" w142 {
      tunnel: w145 -> [w287 w292 w301 w307 w311 _]
      tunnel: [FALSE FALSE FALSE FALSE TRUE TRUE] -> w136
      tunnel: [0.0 ("output") 0.0 ("output") w298 w303 w308 w316] -> w135
      tunnel: [TRUE TRUE TRUE FALSE TRUE TRUE] -> w134
      tunnel: [w282 w288 w297 w304 w308 w316] -> w129
      tunnel: w128 -> [w282 w288 w297 w304 _ w316]
      frame "null", Default {
        n133 = Unbundle By Name(w287) -> ("Loop ID"=w286:i32)
        n134 = call "null.vi"("This Loop ID"=w286) -> ()  [unwired: 2 in]
      }
      frame "wait" {
        n135 = Unbundle By Name(w292) -> ("Loop ID"=w296:i32, "Exit Value"=w295:i32, "Waiting Loop"=w294:i32, "State to Wait For"=w293:i32)
        n136 = call "wait.vi"("State to wait for"=w293, "Waiting Loop ID"=w294, "time (ms)"=w295, "Current Loop ID"=w296) -> ()  [unwired: 1 out]
      }
      frame "driver control" {
        n137 = Unbundle By Name(w301) -> ("Joystick Y"=w299:dbl)
        n138 = call "Joystick Error Filter.vi"("Axis"=w299) -> ("Filtered Axis"=w298:dbl)
      }
      frame "manual override" {
        n139 = Unbundle By Name(w307) -> ("Joystick Y"=w303:dbl)
      }
      frame "auto", "pickup".."load" {
        # "pickup, pass, auto, and load"
        n140 = disable-structure shown="Disabled" {
          disable-tunnel: w311 -> [w315 _]
          disable-tunnel: [w312 _] -> w308
          frame Disabled {
            n141 = Unbundle By Name(w315) -> ("Joystick Z"=w314:dbl, "State"=w313:T31)
            n142 = call "arm control.vi"("State"=w313, "Z Axis (Tuning)"=w314) -> ("setpoint"=w312:dbl)
          }
          frame Enabled {
          }
        }
      }
      frame "hold position" {
        # "previous auto (only for code to use, not driver) setpoint"
      }
    }
    n143 = feedback-in #2(w129) -> ()
    n144 = disable-structure shown="Enabled" {
      disable-tunnel: w125 -> [w165 _]
      frame Enabled {
        n145 = feedback #3() -> (w166:T12)
        n146 = feedback-in #3(w166) -> ()
        n147 = case shown="\"Reverse\"" w165 {
          tunnel: w166 -> [_ w167 w169]
          frame "Off", Default {
          }
          frame "Reverse" {
            n148 = call-poly <vilib>:"WPI_SolenoidSet.vi"("Value"=WPI_SolenoidValue."Reverse", "SolenoidDevRef"=w167) -> ()  [unwired: 8 in, 2 out]
          }
          frame "Forward" {
            n149 = call-poly <vilib>:"WPI_SolenoidSet.vi"("Value"=WPI_SolenoidValue."Forward", "SolenoidDevRef"=w169) -> ()  [unwired: 8 in, 2 out]
          }
        }
      }
      frame Disabled {
      }
    }
    n150 = disable-structure shown="Enabled" {
      disable-tunnel: w136 -> [w183 _]
      disable-tunnel: w135 -> [w182 w193]
      disable-tunnel: w134 -> [w181 _]
      disable-tunnel: [w179 w193] -> w133
      frame Disabled {
        n151 = case shown="True" w183 {
          tunnel: w182 -> [w189 w192]
          tunnel: [w189 w190] -> w180
          frame False {
            # "open loop"
          }
          frame True {
            n152 = call "arm pid.vi"("Setpoint"=w192, "Autotune?"=FALSE) -> ("Output"=w190:dbl)
          }
        }
        n153 = case shown="True" w181 {
          tunnel: w180 -> [w185 w188]
          tunnel: [w185 w187] -> w179
          tunnel: [cluster{"Arm Safety":bool, "Arm Limit":bool} {"Arm Safety"=FALSE, "Arm Limit"=FALSE} ("Input") w186] -> w177
          frame False {
            # "no safety???"
          }
          frame True {
            # "ahhhh safetys..."
            n154 = call "combined arm safety.vi"("Input"=w188) -> ("Safe Output"=w187:dbl, "Safety"=w186:cluster{"Arm Safety":bool, "Arm Limit":bool})  [unwired: 13 in]
          }
        }
        n155 = call "Dash Bools.vi"("Input"=w177, "Menu"=fg_typedef."Set") -> ()  [unwired: 1 out]
      }
      frame Enabled {
      }
    }
    n156 = case shown="True" w132 {
      tunnel: w131 -> [w160 w162]
      tunnel: [w160 w161] -> w130
      frame False {
        # "no safety"
      }
      frame True {
        # "safety (rate limit only)\nbecause there is no \nencoder"
        n157 = call "belt safety.vi"("Input"=w162) -> ("Safe Output"=w161:dbl)
      }
    }
    n158 = disable-structure shown="Enabled" {
      disable-tunnel: w126 -> [w171 _]
      frame Enabled {
        n159 = feedback #4() -> (w172:T12)
        n160 = feedback-in #4(w172) -> ()
        n161 = case shown="\"Forward\"" w171 {
          tunnel: w172 -> [_ w173 w175]
          frame "Off", Default {
          }
          frame "Reverse" {
            n162 = call-poly <vilib>:"WPI_SolenoidSet.vi"("Value"=WPI_SolenoidValue."Forward", "SolenoidDevRef"=w173) -> ()  [unwired: 8 in, 2 out]
          }
          frame "Forward" {
            n163 = call-poly <vilib>:"WPI_SolenoidSet.vi"("Value"=WPI_SolenoidValue."Reverse", "SolenoidDevRef"=w175) -> ()  [unwired: 8 in, 2 out]
          }
        }
      }
      frame Disabled {
      }
    }
    n164 = feedback #5() -> (w138:T4)
    n165 = feedback-in #5(w138) -> ()
    n166 = case shown="True" w141 {
      tunnel: w140 -> [w195 w199]
      tunnel: w139 -> [w194 w198]
      tunnel: w138 -> [w196 w197]
      frame False {
        n167 = call <vilib>:"WPI_RobotDriveMotors.vi"("RightSpeed"=w194, "LeftSpeed"=w195, "RobotDriveDevRef"=w196) -> ()  [unwired: 6 in, 3 out]
      }
      frame True {
        n168 = call-poly <vilib>:"WPI_RobotDriveArcadeDrive.vi"("Y axis value"=w198, "X axis value"=w199, "RobotDriveDevRef"=w197) -> ()  [unwired: 6 in, 3 out]
      }
    }
    n169 = feedback #6() -> (w78:T5)
    n170 = feedback-in #6(w78) -> ()
    n171 = call "loop timer.vi"() -> ("IPS"=→"Main IPS":dbl, "SPI"=w155:u32)  [unwired: 1 in]
    "Main SPI" <- w155
    n172 = call "performance fg.vi"("Menu"=fg_typedef."Get") -> ("Output"=w152:T26)  [unwired: 1 in]
    n173 = Bundle By Name(cluster=w152, "Main mSPI"=w155) -> (w151:T26)
    n174 = disable-structure shown="Enabled" {
      disable-tunnel: w133 -> [w163 _]
      frame Disabled {
        # "(+ or -) raises arm"
        n175 = feedback #7() -> (w164:T5)
        n176 = feedback-in #7(w164) -> ()
        n177 = call <vilib>:"WPI_MotorControlSetOutput.vi"("Output"=w163, "MotorControlDevRef"=w164) -> ()  [unwired: 7 in, 3 out]
      }
      frame Enabled {
      }
    }
    n178 = call <vilib>:"WPI_MotorControlSetOutput.vi"("Output"=w130, "MotorControlDevRef"=w78) -> ()  [unwired: 7 in, 3 out]
    n179 = call "performance fg.vi"("Input"=w151, "Menu"=fg_typedef."Set") -> ()  [unwired: 1 out]
  }
  n180 = Merge Errors("error in", w20, w15, w8, w9, w7, w4) -> (→"error out":errorcluster)
  "error In" <- "error in"
